vi "DQMH-GenNet Get Network Info.vi"(8 "error in (no error)":errorcluster, 11 "Message Queue in":refnum<class "DQMH-GenNet Message Queue.lvclass">) -> (0 "error out":errorcluster, 1 "Port Number":u16, 2 "IP Address":string, 3 "Message Queue out":refnum<class "DQMH-GenNet Message Queue.lvclass">, 4 "Timeout":i32)   [LabVIEW 2014, in "hse-gennet.lvlib" / "DQMH-GenNet Message Queue.lvclass"]
doc: "Gets the network information from the Message Queue"
uses:
  DQMH-GenNet Message Queue.lvclass
  DQMH-GenNet Message Queue.lvclass/DQMH-GenNet Message Queue.ctl
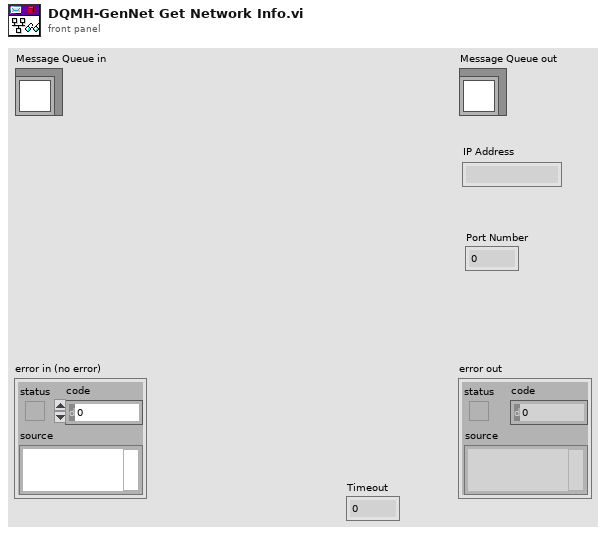
[diagram p1: front panel]
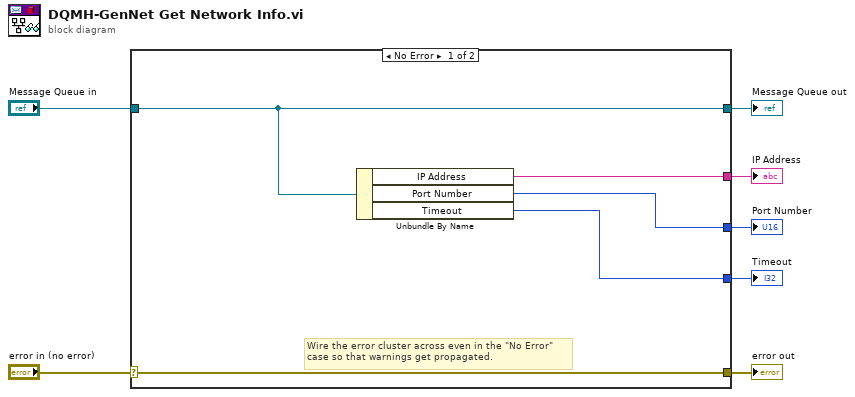
[diagram p0: block diagram]
diagram:
  n1 = case shown="No Error" "error in (no error)" {
    selector: "error in (no error)" -> [w12 w14]
    tunnel: [w12 w14] -> w6
    tunnel: [w11 w13] -> w4
    tunnel: "Message Queue in" -> [w11 w13]
    tunnel: [w10 _] -> w3
    tunnel: [w9 _] -> w2
    tunnel: [w8 _] -> w1
    frame No Error {
      # "Wire the error cluster across even in the \"No Error\"\ncase so that warnings get propagated."
      n2 = Unbundle By Name(w11) -> ("IP Address"=w10:string, "Port Number"=w9:u16, "Timeout"=w8:i32)
    }
    frame Error {
    }
  }
  "error out" <- w6
  "Message Queue out" <- w4
  "IP Address" <- w3
  "Port Number" <- w2
  "Timeout" <- w1
